vi "LPC set control mode.vi"(8 "error in (no error)":errorcluster, 10 "control mode":T1(ring), 11 "VISA resource name":refnum<visa-resource-name>="GPIB0::8::INSTR") -> (0 "error out":errorcluster, 3 "VISA resource name out":refnum<visa-resource-name>)   [LabVIEW 2009, in "Laser Power Controller.lvclass"]
doc: "Sets the control mode (constant power or constant percent transmission) of the LPC (laser power controller)."
uses:
  Laser Power Controller.lvclass
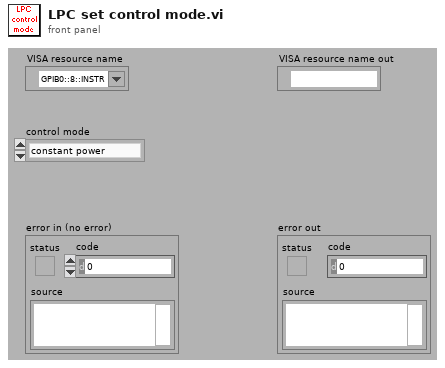
[diagram p1: front panel]
types:
  T1 = enum16{"constant power", "constant transmission"}
  T2 = typedef "Semaphore RefNum" = refnum<k1>
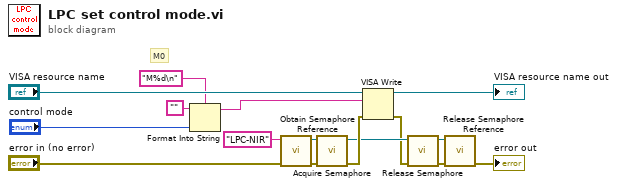
[diagram p0: block diagram]
diagram:
  # "M0"
  n1 = Format Into String(format string="M%d\n", initial string="", "control mode") -> (resulting string=w12:string)  [unwired: 1 in, 1 out]
  n2 = call <vilib>:"Obtain Semaphore Reference.vi"("error in (no error)"="error in (no error)", "name (unnamed)"="LPC-NIR") -> ("error out"=w8:errorcluster, "semaphore"=w7:T2)  [unwired: 1 in, 3 out]
  n3 = call <vilib>:"Acquire Semaphore.vi"("error in (no error)"=w8, "semaphore"=w7) -> ("error out"=w4:errorcluster, "semaphore out"=w3:T2)  [unwired: 1 in, 3 out]
  n4 = VISA Write(VISA resource name="VISA resource name", write buffer=w12, error in (no error)=w4) -> (VISA resource name out=→"VISA resource name out":refnum<visa-resource-name>, error out=w2:errorcluster)  [unwired: 1 out]
  n5 = call <vilib>:"Release Semaphore.vi"("error in (no error)"=w2, "semaphore"=w3) -> ("error out"=w6:errorcluster, "semaphore out"=w5:T2)  [unwired: 4 out]
  n6 = call <vilib>:"Release Semaphore Reference.vi"("error in (no error)"=w6, "semaphore"=w5) -> ("error out"=→"error out":errorcluster)  [unwired: 9 out]
